vi "Util_Trajectory_Absolute_To_Relative.vi"(11 "absTRAJECTORY":T1 {"States"."POSE"."ROTATION"."SIN" format="%13.4f"; "States"."POSE"."ROTATION"."COS" format="%13.4f"; "States"."POSE"."ROTATION"."VALUE" format="%13.4f"; "States"."POSE"."TRANSLATION"."Y" format="%14.3f"; "States"."POSE"."TRANSLATION"."X" format="%14.3f"; "TotalTImeSecs" format="%20.3f"}) -> (3 "outputRelativeTRAJECTORY":T1 {"States"."POSE"."ROTATION"."SIN" format="%13.4f"; "States"."POSE"."ROTATION"."COS" format="%13.4f"; "States"."POSE"."ROTATION"."VALUE" format="%13.4f"; "States"."POSE"."TRANSLATION"."Y" format="%14.3f"; "States"."POSE"."TRANSLATION"."X" format="%14.3f"; "TotalTImeSecs" format="%20.3f"})   [LabVIEW 2019, in "Trajectory_Library.lvlib"]
doc: "Utility function to convert an absolute trajectory to a robot relative trajectory. A robot relative trajectory's initial pose is at X,Y,Ang = 0,0,0"
uses:
  Trajectory_Library.lvlib
  TRAJECTORY.ctl
  TRAJ_STATE.ctl
  POSE2D.ctl
  TRANSLATION2D.ctl
  ROTATION2D.ctl
  Rotation_CreateAngle.vi
  Translation_Create.vi
  Rotation_UnaryMinus.vi
  Translation_RotateBy.vi
  Translation_Minus.vi
  Rotation_Minus.vi
  Rotation_RotateBy.vi
  Rotation_CreateXY.vi
  Util_CalcDist.vi
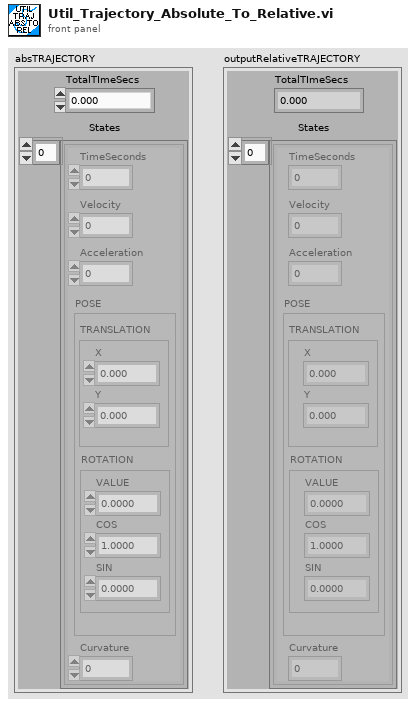
[diagram p1: front panel]
types:
  T1 = typedef "Trajectory_Library.lvlib/TRAJECTORY.ctl" = cluster{"TotalTImeSecs":dbl, "States":T2[]}
  T2 = typedef "Trajectory_Library.lvlib/TRAJ_STATE.ctl" = cluster{"TimeSeconds":dbl, "Velocity":dbl, "Acceleration":dbl, "POSE":T3, "Curvature":dbl}
  T3 = typedef "Trajectory_Library.lvlib/POSE2D.ctl" = cluster{"TRANSLATION":T4, "ROTATION":T5}
  T4 = typedef "Trajectory_Library.lvlib/TRANSLATION2D.ctl" = cluster{"X":dbl, "Y":dbl}
  T5 = typedef "Trajectory_Library.lvlib/ROTATION2D.ctl" = cluster{"VALUE":dbl, "COS":dbl, "SIN":dbl}
  T6 = typedef "Trajectory_Library.lvlib/TRANSFORM2D.ctl" = cluster{"TRANSLATION":T4, "ROTATION":T5}
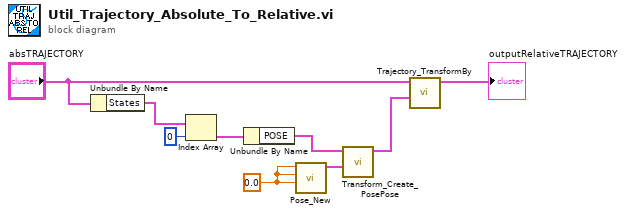
[diagram p0: block diagram]
diagram:
  w5 = 0.0 ("X")
  n1 = Unbundle By Name("absTRAJECTORY") -> ("States"=w9:T2[])
  n2 = Index Array(array=w9, index=0) -> (element=w2:T2)
  n3 = Unbundle By Name(w2) -> ("POSE"=w4:T3)
  n4 = call "Pose_New.vi"("Heading"=w5, "Y"=w5, "X"=w5) -> ("out POSe"=w6:T3)  [unwired: 8 in]
  n5 = call "Transform_Create_PosePose.vi"("last POSE"=w6, "initial POSE"=w4) -> ("TRANSFORM"=w7:T6)  [unwired: 9 in]
  n6 = call "Trajectory_TransformBy.vi"("TRANSFORM"=w7, "InputTRAJECTORY"="absTRAJECTORY") -> ("outputTRAJECTORY"=→"outputRelativeTRAJECTORY":T1)  [unwired: 9 in]
